vi "双串口例程.vi"() -> ()   [LabVIEW 2013]
doc: "本范例根据用户指示，对串口执行读写操作。范例运行时可按下“写入”或“读取”按钮，以及修改“读数”。\n\n设置的串口参数必须匹配连接仪器或设备的参数。本范例中，“读数”参数可指定串口读取的字节数。如端口字节超过指定的字节数，超出部分将不会被读取。如端口字节数少于指定的字节数，将返回超时错误。\n\n本范例可扩展流控制选项以包括XON和XOFF，从而允许用户选择控制字符。同时，用户可启用或禁用中止符。部分设备需要通过终止符确定命令字符串的结束位置。部分设备将发送终止符以说明待读取数据的末端。本范例演示了缓冲区中检测到终止符时，结束“读取”操作或添加终止符至“写入”数据末端的方法。"
uses:
  E:/National Instruments/LabVIEW 2013/examples/Instrument IO/Serial/support/Serial - Settings.ctl
  <vilib>/Instr/_visa.llb/VISA Configure Serial Port (Instr).vi
panel:
  out "这是车头X坐标，其他同理，看通讯协议":u8
  in  "右转速给这里":u8
  in  "左转速给这里":u8
  in  "方向给这里":u8
  out "坐标在这里边":u8[](array[numeric])
  in  "读取":bool
  out "响应":string
  in  "读数":u32=1000
  in  "VISA资源名称 读取":refnum<visa-resource-name>="COM1"
  in  "串口设置 读取":T1={"波特率"=9600, "数据比特"=8, "奇偶"=enum."None", "停止位"=10, "流控制"=0} {"流控制" items=["无"=0, "XON/XOFF"=1, "RTS/CTS"=2, "DTR/DSR"=4]; "停止位" items=["1.0"=10, "1.5"=15, "2.0"=20]; "数据比特" min=5 max=8 step=1; "波特率" items=["75"=75, "110"=110, "134"=134, "150"=150, "300"=300, "600"=600, "1200"=1200, "1800"=1800, "2400"=2400, "4800"=4800, "7200"=7200, "9600"=9600, "14400"=14400, "19200"=19200, "28800"=28800, "38400"=38400, "56000"=56000, "57600"=57600, "115200"=115200, "128000"=128000, "230400"=230400]}
  in  "终止符时结束读取？":bool=TRUE
  in  "终止符":u8=10 format="%.0x"
  in  "终止符时结束写入？":bool=TRUE
  in  "停止":bool
  out "命令":string="*IDN?"
  in  "写入":bool
  in  "串口设置 写入":T1={"波特率"=9600, "数据比特"=8, "奇偶"=enum."None", "停止位"=10, "流控制"=0} {"流控制" items=["无"=0, "XON/XOFF"=1, "RTS/CTS"=2, "DTR/DSR"=4]; "停止位" items=["1.0"=10, "1.5"=15, "2.0"=20]; "数据比特" min=5 max=8 step=1; "波特率" items=["75"=75, "110"=110, "134"=134, "150"=150, "300"=300, "600"=600, "1200"=1200, "1800"=1800, "2400"=2400, "4800"=4800, "7200"=7200, "9600"=9600, "14400"=14400, "19200"=19200, "28800"=28800, "38400"=38400, "56000"=56000, "57600"=57600, "115200"=115200, "128000"=128000, "230400"=230400]}
  in  "VISA资源名称 写入":refnum<visa-resource-name>="COM1"
  # "概述：演示在循环中使用VISA函数连续写入命令至串口仪器或从串口仪器读取响应。\n要求：NI-VISA驱动程序\n操作步骤：\n1. 运行VI。\n2. 指定命令并单击写入按钮。\n3. 单击读取按钮读取响应。\n4. 单击停止按钮停止VI。"
  # "0xA相当于'\\n'字符，为换行符。"
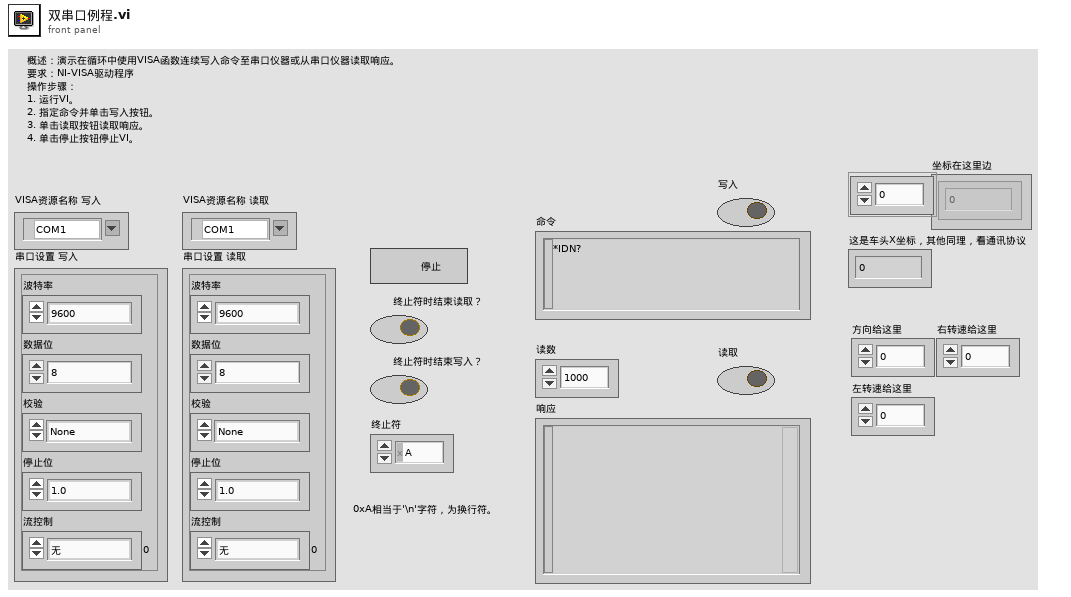
[diagram p1: front panel]
types:
  T1 = typedef "Serial - Settings.ctl" = cluster{"波特率":u32, "数据比特":u16, "奇偶":enum16{"None", "Odd", "Even", "Mark", "Space"}, "停止位":u16, "流控制":u16}
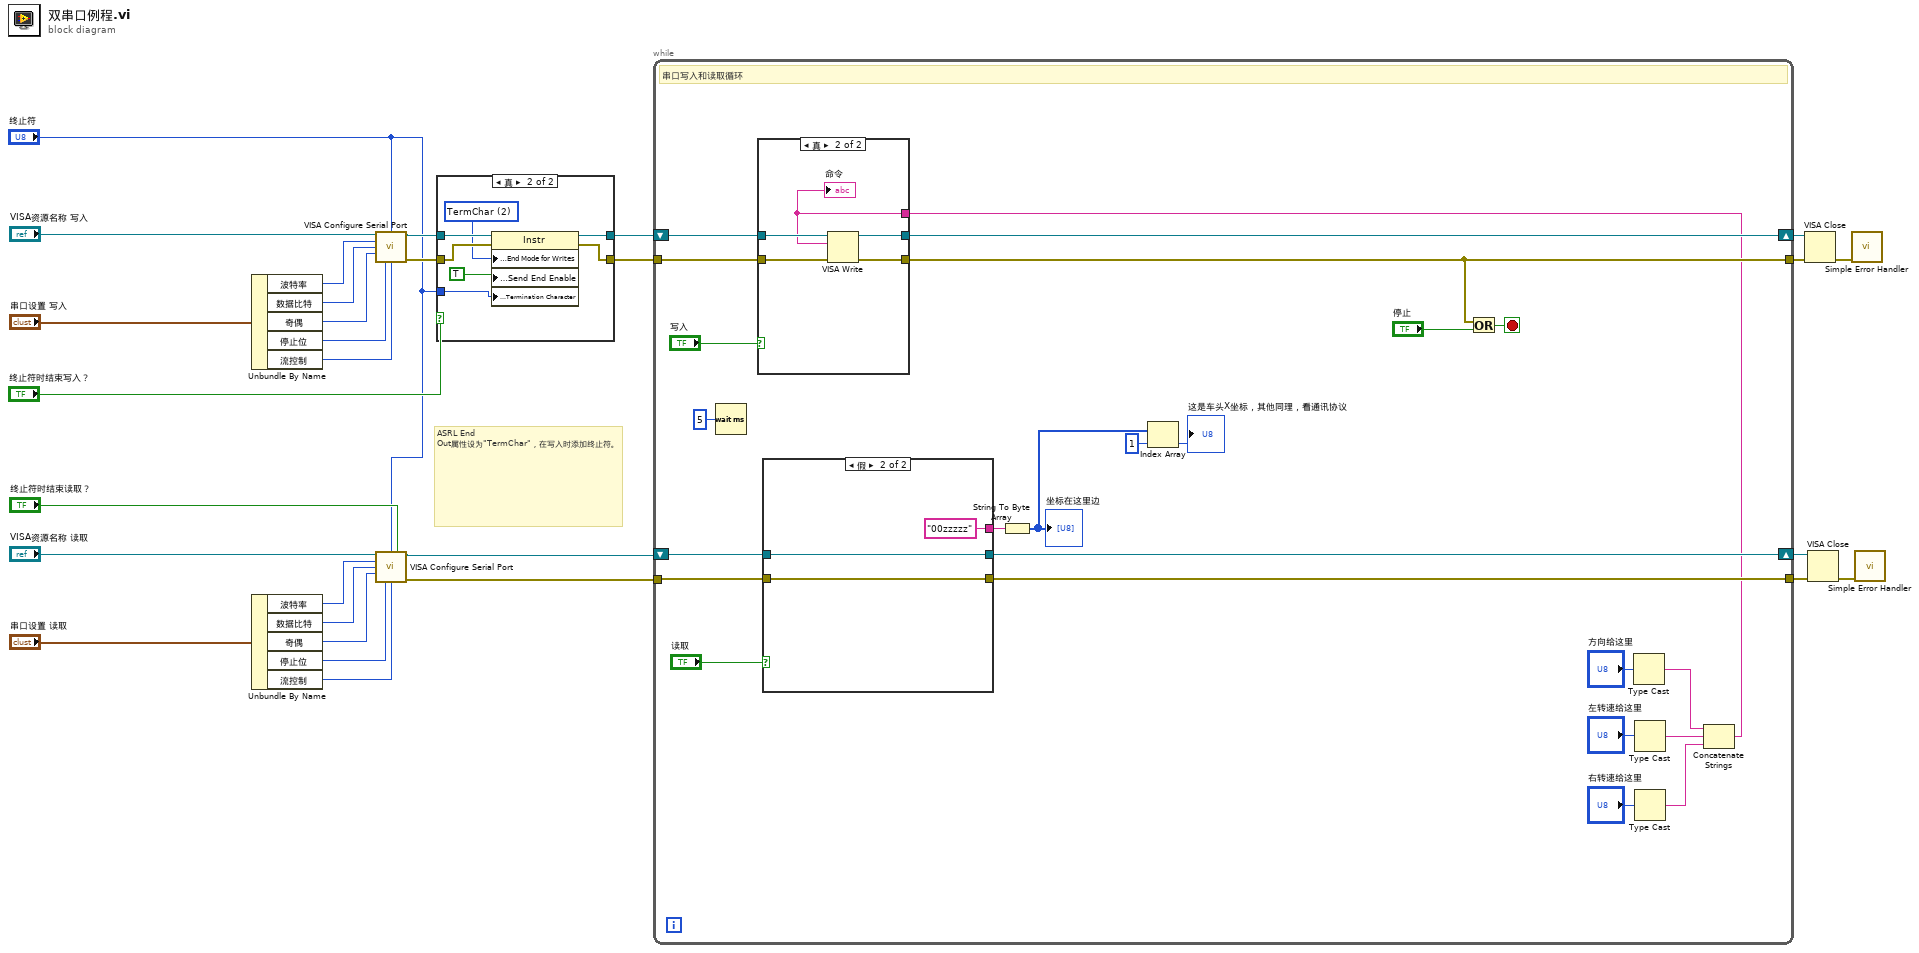
[diagram p0: block diagram]
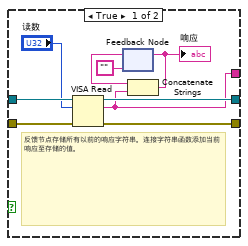
[diagram p3: hidden frame]
diagram:
  # "ASRL End Out属性设为\"TermChar\"，在写入时添加终止符。"
  n1 = Unbundle By Name("串口设置 写入") -> ("波特率"=w25:u32, "数据比特"=w26:u16, "奇偶"=w27:enum16{"None", "Odd", "Even", "Mark", "Space"}, "停止位"=w28:u16, "流控制"=w21:u16)
  n2 = Unbundle By Name("串口设置 读取") -> ("波特率"=w13:u32, "数据比特"=w14:u16, "奇偶"=w15:enum16{"None", "Odd", "Even", "Mark", "Space"}, "停止位"=w16:u16, "流控制"=w9:u16)
  n3 = call-poly "VISA Configure Serial Port"("VISA resource name"="VISA资源名称 写入", "termination char\n(0xA = '\\n' = LF)"="终止符", "baud rate (9600)"=w25, "data bits (8)"=w26, "parity (0:none)"=w27, "stop bits (10: 1 bit)"=w28, "flow control (0:none)"=w21) -> ("VISA resource name out"=w7:refnum<visa-resource-name>, "error out"=w6:errorcluster)  [unwired: 3 in, 4 out]
  n4 = call-poly "VISA Configure Serial Port"("VISA resource name"="VISA资源名称 读取", "termination char\n(0xA = '\\n' = LF)"="终止符", "Enable Termination\nChar (T)"="终止符时结束读取？", "baud rate (9600)"=w13, "data bits (8)"=w14, "parity (0:none)"=w15, "stop bits (10: 1 bit)"=w16, "flow control (0:none)"=w9) -> ("VISA resource name out"=w3:refnum<visa-resource-name>, "error out"=w2:errorcluster)  [unwired: 2 in, 4 out]
  n5 = case shown="真" "终止符时结束写入？" {
    tunnel: w7 -> [w30 w38]
    tunnel: w6 -> [w31 w37]
    tunnel: [w30 w36] -> w19
    tunnel: [w31 w35] -> w20
    tunnel: "终止符" -> [_ w33]
    frame False {
    }
    frame True {
      w34 = u16 2 items=["None", "LastBit", "TermChar", "Break"] ("Serial Settings:Serial End Mode for Writes")
      n6 = property class="Instr"(reference=w38, error in=w37, "Serial Settings:End Mode for Writes"=w34, "Message Based Settings:Send End Enable"=TRUE, "Message Based Settings:Termination Character"=w33) -> (reference out=w36:refnum<visa-resource-name>, error out=w35:errorcluster)
    }
  }
  n7 = while {
    shift-right: [w52] -> w22
    shift-left: w19 -> [w62]
    tunnel: w20 -> [w61]
    tunnel: w2 -> [w53]
    shift-right: [w55] -> w8
    shift-left: w3 -> [w54]
    tunnel: [w51] -> w5
    tunnel: [w50] -> w4
    stop <- w59 stop-if-true
    # "串口写入和读取循环"
    n8 = Wait (ms)(milliseconds to wait=u32 5) -> ()  [unwired: 1 out]
    n9 = case shown="假" "读取" {
      tunnel: [w69 w74] -> w55
      tunnel: w54 -> [w71 w74]
      tunnel: [w67 w73] -> w50
      tunnel: w53 -> [w70 w73]
      tunnel: [w63 "00zzzzz" ("read buffer")] -> w46
      frame True {
        # "反馈节点存储所有以前的响应字符串。连接字符串函数添加当前响应至存储的值。"
        n10 = VISA Read(VISA resource name=w71, byte count="读数", error in (no error)=w70) -> (VISA resource name out=w69:refnum<visa-resource-name>, read buffer=w63:string, error out=w67:errorcluster)  [unwired: 1 out]
        n11 = feedback #1("") -> (w66:string)
        n12 = Concatenate Strings(w66, w63) -> (w64:string)
        "响应" <- w64
        n13 = feedback-in #1(w64) -> ()
      }
      frame False {
      }
    }
    n14 = String To Byte Array(string=w46) -> (unsigned byte array=w41:u8[])
    "坐标在这里边" <- w41
    n15 = Index Array(array=w41, index=1 ("索引")) -> (element=→"这是车头X坐标，其他同理，看通讯协议":u8)
    n16 = Type Cast(x="方向给这里") -> (*(type *) &x=w49:string)  [unwired: 1 in]
    n17 = Type Cast(x="左转速给这里") -> (*(type *) &x=w48:string)  [unwired: 1 in]
    n18 = Type Cast(x="右转速给这里") -> (*(type *) &x=w47:string)  [unwired: 1 in]
    n19 = Concatenate Strings(w49, w48, w47) -> (w45:string)
    n20 = case shown="真" "写入" {
      tunnel: w62 -> [w76 w81]
      tunnel: w61 -> [w75 w80]
      tunnel: [w76 w79] -> w52
      tunnel: [w75 w78] -> w51
      tunnel: w45 -> [_ w77]
      frame False {
      }
      frame True {
        n21 = VISA Write(VISA resource name=w81, write buffer=w77, error in (no error)=w80) -> (VISA resource name out=w79:refnum<visa-resource-name>, error out=w78:errorcluster)  [unwired: 1 out]
        "命令" <- w77
      }
    }
    n22 = Or(x=w51, y="停止") -> (x .or. y?=w59:bool)
  }
  n23 = VISA Close(VISA resource name=w22, error in (no error)=w5) -> (error out=w23:errorcluster)
  n24 = VISA Close(VISA resource name=w8, error in (no error)=w4) -> (error out=w10:errorcluster)
  n25 = call <vilib>:"Simple Error Handler.vi"("error in (no error)"=w23) -> ()  [unwired: 1 in, 8 out]
  n26 = call <vilib>:"Simple Error Handler.vi"("error in (no error)"=w10) -> ()  [unwired: 1 in, 8 out]
